vi "ClearReplyCode.vi"(1 "SRV In":string="169.254.0.10") -> (0 "SRV Out":string="169.254.0.10")   [LabVIEW 2009]
panel:
  # "This LabVIEW item is deprecated.\n\nIt is believed to be unused and will be removed in a future version of SRV."
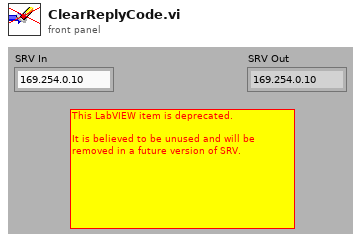
[diagram p1: front panel]
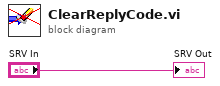
[diagram p0: block diagram]
diagram:
  "SRV Out" <- "SRV In"
